vi "AlliGator Creat X & Y Coordinate Arrays.vi"(9 "Y":i32, 11 "X":i32) -> (1 "Y Array":i32[](array[numeric]), 3 "X array":i32[](array[numeric]))   [LabVIEW 2021, in "AlliGator Decay Fit Parameter Map.lvlib"]
doc: "Creates two arrays used in Load Fit Data (Map) mat File,vi to insert pixel coordinates in front of fit parameters."
uses:
  AlliGator Decay Fit Parameter Map.lvlib
  Arrays/Arrays.lvlib
panel:
  # "see the License on the block diagram (Ctrl+E or Window:Show Block Diagram)"
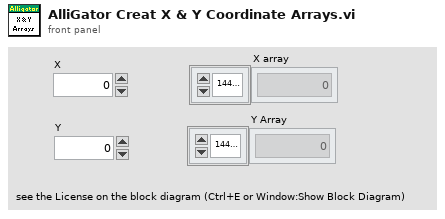
[diagram p1: front panel]
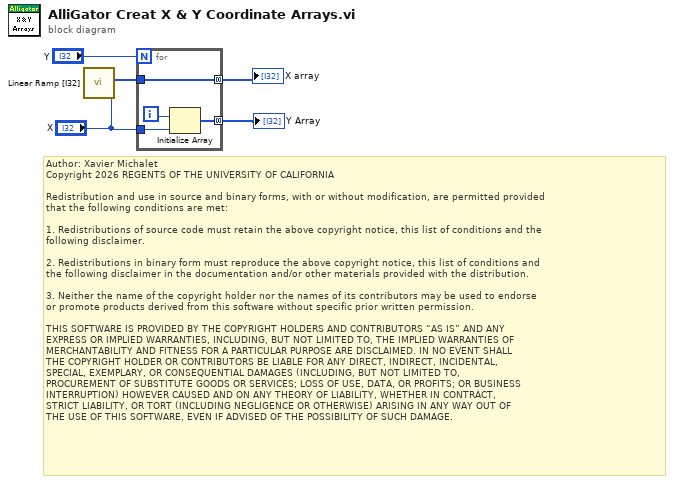
[diagram p0: block diagram]
diagram:
  # "Author: Xavier Michalet\nCopyright 2026 REGENTS OF THE UNIVERSITY OF CALIFORNIA\n\nRedistribution and use in source and binary forms, with or without modification, are permitted provided\nthat the following conditions are met:\n\n1. Redistributions of source code must retain the above copyright notice, this list of conditions and the\nfollowing disclaimer.\n\n2. Redistributions in binary form must reproduce the above copyright notice, this list of conditions and\nthe following disclaimer in the documentation and/or other materials provided with the distribution.\n\n3. Neither the name of the copyright holder nor the names of its contributors may be used to endorse \nor promote products derived from this software without specific prior written permission.\n\nTHIS SOFTWARE IS PROVIDED BY THE COPYRIGHT HOLDERS AND CONTRIBUTORS “AS IS” AND ANY \nEXPRESS OR IMPLIED WARRANTIES, INCLUDING, BUT NOT LIMITED TO, THE IMPLIED WARRANTIES OF\nMERCHANTABILITY AND FITNESS FOR A PARTICULAR PURPOSE ARE DISCLAIMED. IN NO EVENT SHALL\nTHE COPYRIGHT HOLDER OR CONTRIBUTORS BE LIABLE FOR ANY DIRECT, INDIRECT, INCIDENTAL, \nSPECIAL, EXEMPLARY, OR CONSEQUENTIAL DAMAGES (INCLUDING, BUT NOT LIMITED TO, \nPROCUREMENT OF SUBSTITUTE GOODS OR SERVICES; LOSS OF USE, DATA, OR PROFITS; OR BUSINESS\nINTERRUPTION) HOWEVER CAUSED AND ON ANY THEORY OF LIABILITY, WHETHER IN CONTRACT, \nSTRICT LIABILITY, OR TORT (INCLUDING NEGLIGENCE OR OTHERWISE) ARISING IN ANY WAY OUT OF\nTHE USE OF THIS SOFTWARE, EVEN IF ADVISED OF THE POSSIBILITY OF SUCH DAMAGE."
  n1 = call "Linear Ramp [I32].vi"("# Elements"="X") -> ("Ramp"=w5:i32[])  [unwired: 8 in]
  n2 = for {
    N: "Y" -> [_]
    tunnel: [w9] -> w4 mode=concatenating
    tunnel: w5 -> [w9]
    tunnel: "X" -> [w7]
    tunnel: [w6] -> w1 mode=concatenating
    i -> [w8]
    n3 = Initialize Array(w8, w7) -> (w6:i32[])
  }
  "Y Array" <- w1
  "X array" <- w4
